vi "post_mlt.vi"   [LabVIEW 2012]
uses:
  <vilib>/addons/internet/NI_InternetTK_Core_VIs.lvlib
types:
  T1 = typedef "CGI Connection Info.ctl" = cluster{"name":string, "type":T2, "session":T3}
  T2 = typedef "CGI Request Type.ctl" = enum16{"cgi", ".spool first", ".spool", ".spool last"}
  T3 = typedef "HTTP Session.ctl" = refnum<k1>
  T4 = typedef "NI_FTP.lvlib/Keyed Array.ctl" = cluster{"keys":string[], "values":string[]}
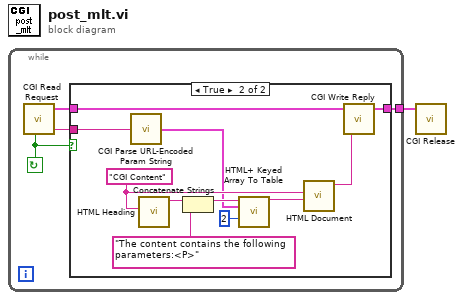
[diagram p0: block diagram]
diagram:
  n1 = while {
    tunnel: [w4] -> w1
    stop <- w3 continue-if-true
    n2 = call <vilib>:"CGI Read Request.vi"() -> ("valid request?"=w3:bool, "cgi connection info"=w5:T1, "content"=w2:string)  [unwired: 4 in, 1 out]
    n3 = case shown="True" w3 {
      tunnel: [w6 w17] -> w4
      tunnel: w5 -> [w6 w16]
      tunnel: w2 -> [_ w8]
      frame False {
      }
      frame True {
        w14 = "CGI Content" ("heading")
        n4 = call <vilib>:"CGI Parse URL-Encoded Param String.vi"("url-encoded param string"=w8) -> ("params"=w7:T4)
        n5 = call <vilib>:"HTML Heading.vi"("heading"=w14) -> ("HTML out"=w13:string)  [unwired: 10 in]
        n6 = Concatenate Strings(w13, "The content contains the following parameters:<P>" ("label")) -> (w12:string)
        n7 = call <vilib>:"HTML+ Keyed Array To Table.vi"("HTML in"=w12, "keyed array"=w7, "border width (default)"=2) -> ("HTML out"=w10:string)  [unwired: 12 in]
        n8 = call <vilib>:"HTML Document.vi"("document body"=w10, "document title"=w14) -> ("HTML Document"=w15:string)  [unwired: 9 in]
        n9 = call <vilib>:"CGI Write Reply.vi"("content"=w15, "cgi connection info"=w16) -> ("cgi connection info out"=w17:T1)  [unwired: 3 in]
      }
    }
  }
  n10 = call <vilib>:"CGI Release.vi"("cgi connection info"=w1) -> ()  [unwired: 5 in]
